vi "Generate Nonce.vi"() -> (2 "nonce":string)   [LabVIEW 2011, in "i3-oauth.lvlib"]
doc: "Generates a sudo-random number for use as an OAuth nonce value."
uses:
  i3-oauth.lvlib
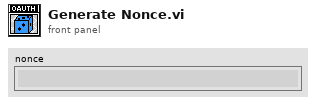
[diagram p1: front panel]
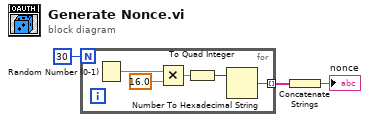
[diagram p0: block diagram]
diagram:
  n1 = for {
    N: 30 -> [_]
    tunnel: [w4] -> w2 mode=indexing
    n2 = Random Number (0-1)() -> (number: 0 to 1=w8:dbl)
    n3 = Multiply(x=w8, y=16.0) -> (x*y=w6:dbl)
    n4 = To Quad Integer(1:w6) -> (0:w5:i64)
    n5 = Number To Hexadecimal String(2:w5) -> (0:w4:string)  [unwired: 1 in]
  }
  n6 = Concatenate Strings(w2) -> (→"nonce":string)
